vi "Batería electrónica (Main aplicación).vi"() -> ()   [LabVIEW 2015]
doc: "Este Vi contiene la máquina de estados necesaria para simular una batería electrónica, utilizando librerías DAQ y Arduino para recibir señales."
uses:
  <vilib>/DAQmx/read.llb/DAQmx Read (Analog DBL 1Chan 1Samp).vi
  <vilib>/DAQmx/create/channels.llb/DAQmx Create Channel (AI-Voltage-Basic).vi
  <vilib>/sound2/lvsound2.llb/Sound Output Write (DBL).vi
  <vilib>/DAQmx/miscellaneous.llb/DAQmx Fill In Error Info.vi
panel:
  in  "Stop Button":bool
  # "Batería Electrónica\nIICO UASLP"
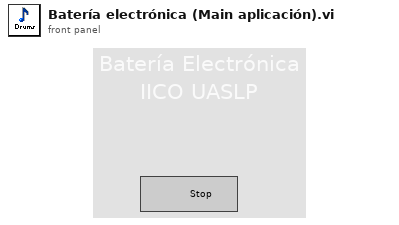
[diagram p1: front panel]
types:
  T1 = typedef "Control para máquina de estados.ctl" = enum16{"Bombo", "Medium Tom", "High Tom", "Hi-Hat ", "Tarola", "Tom de Piso", "Ride", "Crash"}
  T2 = typedef "Sound Output Task ID.ctl" = u32
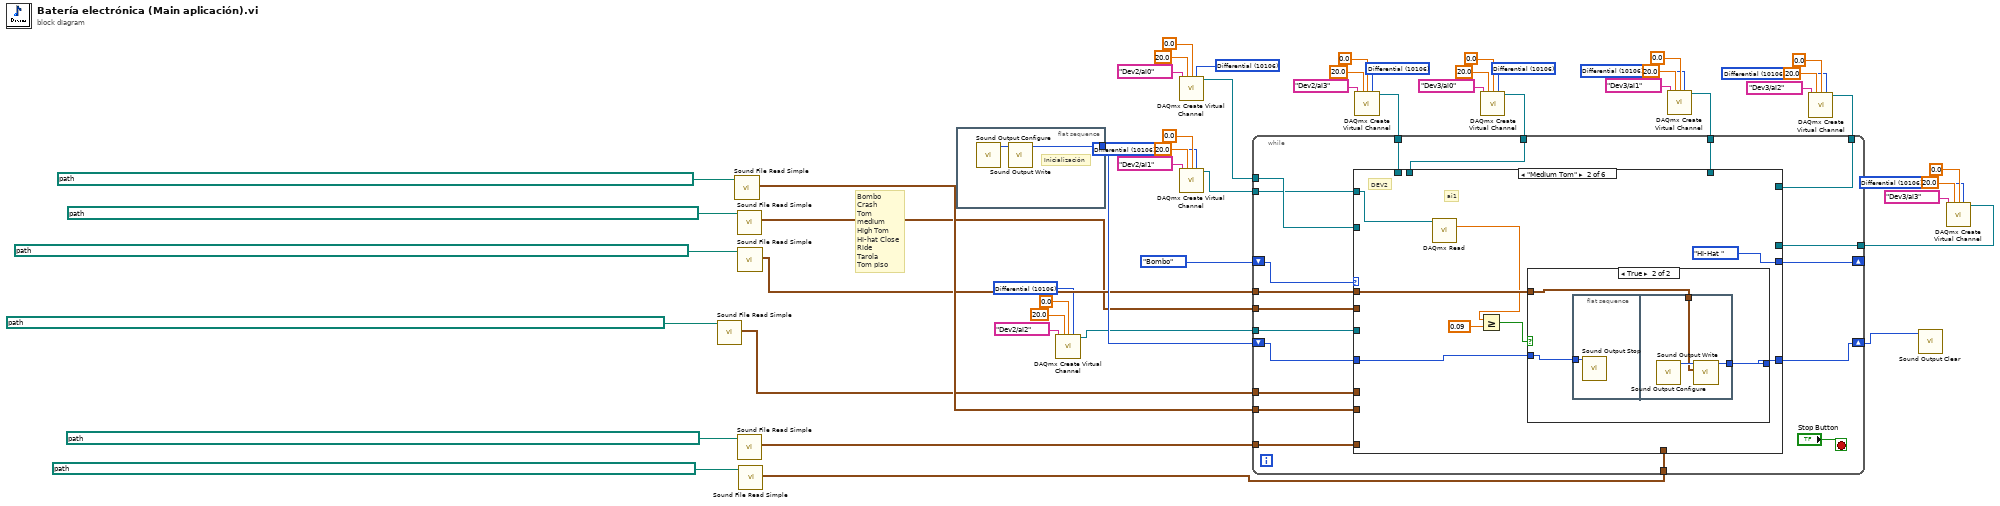
[diagram p0: block diagram]
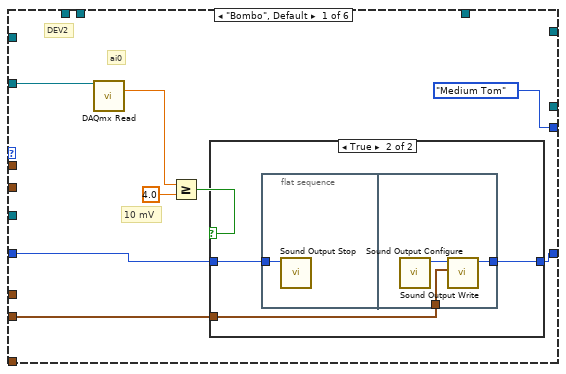
[diagram p2: hidden frame]
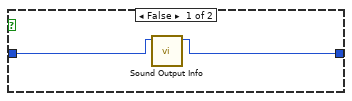
[diagram p3: hidden frame]
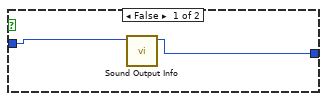
[diagram p4: hidden frame]
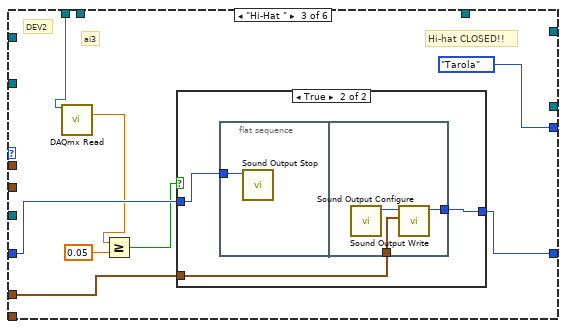
[diagram p5: hidden frame]
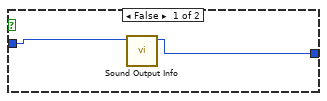
[diagram p6: hidden frame]
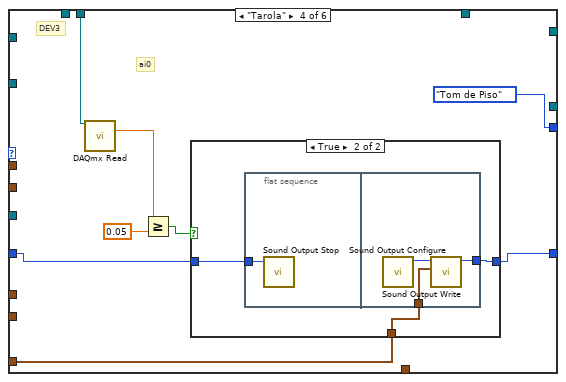
[diagram p7: hidden frame]
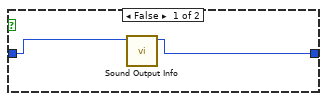
[diagram p8: hidden frame]
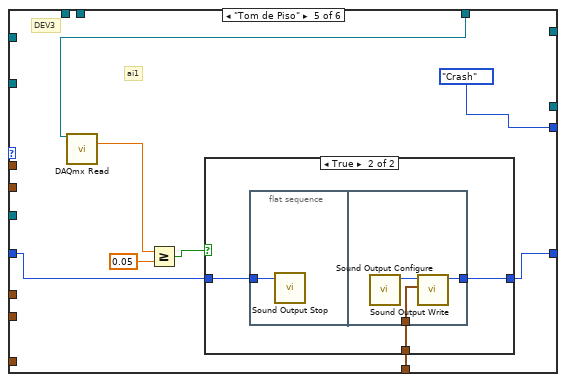
[diagram p9: hidden frame]
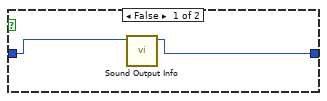
[diagram p10: hidden frame]
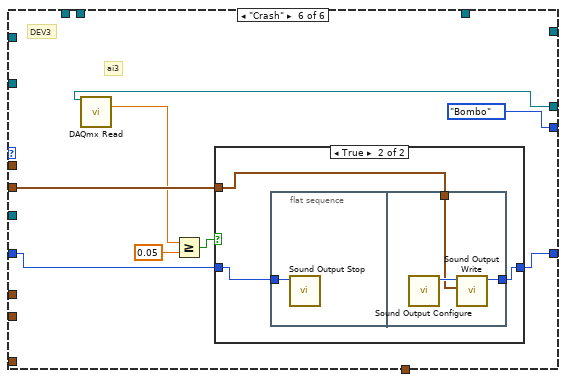
[diagram p11: hidden frame]
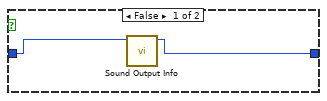
[diagram p12: hidden frame]
diagram:
  w2 = 10106 items=["Default"=-1, "RSE"=10083, "NRSE"=10078, "Differential"=10106, "Pseudodifferential"=12529] ("input terminal configuration")
  w6 = 10106 items=["Default"=-1, "RSE"=10083, "NRSE"=10078, "Differential"=10106, "Pseudodifferential"=12529] ("input terminal configuration")
  w8 = 10106 items=["Default"=-1, "RSE"=10083, "NRSE"=10078, "Differential"=10106, "Pseudodifferential"=12529] ("input terminal configuration")
  w13 = 10106 items=["Default"=-1, "RSE"=10083, "NRSE"=10078, "Differential"=10106, "Pseudodifferential"=12529] ("input terminal configuration")
  w18 = 10106 items=["Default"=-1, "RSE"=10083, "NRSE"=10078, "Differential"=10106, "Pseudodifferential"=12529] ("input terminal configuration")
  w22 = 10106 items=["Default"=-1, "RSE"=10083, "NRSE"=10078, "Differential"=10106, "Pseudodifferential"=12529] ("input terminal configuration")
  w23 = 10106 items=["Default"=-1, "RSE"=10083, "NRSE"=10078, "Differential"=10106, "Pseudodifferential"=12529] ("input terminal configuration")
  w24 = 10106 items=["Default"=-1, "RSE"=10083, "NRSE"=10078, "Differential"=10106, "Pseudodifferential"=12529] ("input terminal configuration")
  # "Bombo\nCrash\nTom medium\nHigh Tom\nHi-hat Close\nRide\nTarola\nTom piso"
  n1 = call <vilib>:"Sound File Read Simple.vi"("path"=path "C:/Users/user/Dropbox/INGENIERÍA FÍSICA/6to. Semestre/Laboratorio Ing Física 2 (Labview)/PROYECTO FINAL/Programa Final/seleccion final de samples/hi hat closed.wav") -> ("data"=w50:waveform(dbl)[])  [unwired: 7 in, 3 out]
  n2 = call <vilib>:"Sound File Read Simple.vi"("path"=path "C:/Users/user/Dropbox/INGENIERÍA FÍSICA/6to. Semestre/Laboratorio Ing Física 2 (Labview)/PROYECTO FINAL/Programa Final/seleccion final de samples/Bombo.wav") -> ("data"=w52:waveform(dbl)[])  [unwired: 7 in, 3 out]
  n3 = call <vilib>:"Sound File Read Simple.vi"("path"=path "C:/Users/user/Dropbox/INGENIERÍA FÍSICA/6to. Semestre/Laboratorio Ing Física 2 (Labview)/PROYECTO FINAL/Programa Final/seleccion final de samples/crash.wav") -> ("data"=w47:waveform(dbl)[])  [unwired: 7 in, 3 out]
  n4 = call <vilib>:"Sound File Read Simple.vi"("path"=path "C:/Users/user/Dropbox/INGENIERÍA FÍSICA/6to. Semestre/Laboratorio Ing Física 2 (Labview)/PROYECTO FINAL/Programa Final/seleccion final de samples/tarola.wav") -> ("data"=w49:waveform(dbl)[])  [unwired: 7 in, 3 out]
  n5 = call <vilib>:"Sound File Read Simple.vi"("path"=path "C:/Users/user/Dropbox/INGENIERÍA FÍSICA/6to. Semestre/Laboratorio Ing Física 2 (Labview)/PROYECTO FINAL/Programa Final/seleccion final de samples/tom medium final.wav") -> ("data"=w51:waveform(dbl)[])  [unwired: 7 in, 3 out]
  n6 = call <vilib>:"Sound File Read Simple.vi"("path"=path "C:/Users/user/Dropbox/INGENIERÍA FÍSICA/6to. Semestre/Laboratorio Ing Física 2 (Labview)/PROYECTO FINAL/Programa Final/seleccion final de samples/tom piso.wav") -> ("data"=w48:waveform(dbl)[])  [unwired: 7 in, 3 out]
  n7 = flat-sequence {
    tunnel: [w56] -> w54
    frame #0 {
      # "Inicialización"
      n8 = call <vilib>:"Sound Output Configure.vi"() -> ("task ID"=w57:T2)  [unwired: 10 in, 1 out]
      n9 = call-poly <vilib>:"Sound Output Write.vi"("task ID"=w57) -> ("task ID out"=w56:T2)  [unwired: 9 in, 1 out]
    }
  }
  n10 = call-poly <vilib>:"DAQmx Create Virtual Channel.vi"("maximum value"=20.0, "minimum value"=0.0, "input terminal configuration"=w6, "physical channels"=tag "Dev2/ai2") -> ("task out"=w29:refnum<k21>)  [unwired: 10 in, 1 out]
  n11 = call-poly <vilib>:"DAQmx Create Virtual Channel.vi"("maximum value"=20.0, "minimum value"=0.0, "input terminal configuration"=w23, "physical channels"=tag "Dev2/ai0") -> ("task out"=w39:refnum<k21>)  [unwired: 10 in, 1 out]
  n12 = call-poly <vilib>:"DAQmx Create Virtual Channel.vi"("maximum value"=20.0, "minimum value"=0.0, "input terminal configuration"=w22, "physical channels"=tag "Dev2/ai1") -> ("task out"=w33:refnum<k21>)  [unwired: 10 in, 1 out]
  n13 = call-poly <vilib>:"DAQmx Create Virtual Channel.vi"("maximum value"=20.0, "minimum value"=0.0, "input terminal configuration"=w24, "physical channels"=tag "Dev2/ai3") -> ("task out"=w25:refnum<k21>)  [unwired: 10 in, 1 out]
  n14 = call-poly <vilib>:"DAQmx Create Virtual Channel.vi"("maximum value"=20.0, "minimum value"=0.0, "input terminal configuration"=w18, "physical channels"=tag "Dev3/ai0") -> ("task out"=w17:refnum<k21>)  [unwired: 10 in, 1 out]
  n15 = call-poly <vilib>:"DAQmx Create Virtual Channel.vi"("maximum value"=20.0, "minimum value"=0.0, "input terminal configuration"=w13, "physical channels"=tag "Dev3/ai1") -> ("task out"=w12:refnum<k21>)  [unwired: 10 in, 1 out]
  n16 = call-poly <vilib>:"DAQmx Create Virtual Channel.vi"("maximum value"=20.0, "minimum value"=0.0, "input terminal configuration"=w8, "physical channels"=tag "Dev3/ai2") -> ("task out"=w7:refnum<k21>)  [unwired: 10 in, 1 out]
  n17 = call-poly <vilib>:"DAQmx Create Virtual Channel.vi"("maximum value"=20.0, "minimum value"=0.0, "input terminal configuration"=w2, "physical channels"=tag "Dev3/ai3") -> ("task out"=w1:refnum<k21>)  [unwired: 10 in, 1 out]
  n18 = while {
    shift-right: [w74] -> _
    shift-left: Control_para_máquina_de_estados."Bombo" -> [w75]
    shift-right: [w73] -> w53
    shift-left: w54 -> [w72]
    tunnel: w52 -> [w71]
    tunnel: w51 -> [w70]
    tunnel: w50 -> [w69]
    tunnel: w49 -> [w68]
    tunnel: w48 -> [w67]
    tunnel: w47 -> [w66]
    tunnel: w39 -> [w65]
    tunnel: w33 -> [w64]
    tunnel: w29 -> [w63]
    tunnel: w25 -> [w62]
    tunnel: w17 -> [w61]
    tunnel: w12 -> [w60]
    tunnel: w7 -> [w59]
    tunnel: w1 -> [w58]
    stop <- "Stop Button" stop-if-true
    n19 = case shown="\"Medium Tom\"" w75 {
      tunnel: [Control_para_máquina_de_estados."Medium Tom" Control_para_máquina_de_estados."Hi-Hat " Control_para_máquina_de_estados."Tarola" Control_para_máquina_de_estados."Tom de Piso" Control_para_máquina_de_estados."Crash" Control_para_máquina_de_estados."Bombo"] -> w74
      tunnel: [w83 w99 w114 w134 w150 w167] -> w73
      tunnel: w72 -> [w82 w100 w116 w133 w151 w168]
      tunnel: w71 -> [w81 _ _ _ _ _]
      tunnel: w70 -> [_ w98 _ _ _ _]
      tunnel: w69 -> [_ _ w113 _ _ _]
      tunnel: w68 -> [_ _ _ w132 _ _]
      tunnel: w67 -> [_ _ _ _ w149 _]
      tunnel: w66 -> [_ _ _ _ _ w166]
      tunnel: w65 -> [w78 _ _ _ _ _]
      tunnel: w64 -> [_ w94 _ _ _ _]
      tunnel: w63 -> [_ _ _ _ _ _]
      tunnel: w62 -> [_ _ w111 _ _ _]
      tunnel: w61 -> [_ _ _ w128 _ _]
      tunnel: w60 -> [_ _ _ _ w145 _]
      tunnel: w59 -> [_ _ _ _ _ _]
      tunnel: w58 -> [_ _ _ _ _ w163]
      frame "Bombo", Default {
        # "10 mV"
        # "DEV2"
        # "ai0"
        n20 = call-poly <vilib>:"DAQmx Read.vi"("task/channels in"=w78) -> ("data"=w77:dbl)  [unwired: 12 in, 2 out]
        n21 = Greater Or Equal?(x=w77, y=4.0) -> (x >= y?=w79:bool)
        n22 = case shown="True" w79 {
          tunnel: [w85 w89] -> w83
          tunnel: w82 -> [w86 w87]
          tunnel: w81 -> [_ w88]
          frame False {
            n23 = call <vilib>:"Sound Output Info.vi"("task ID"=w86) -> ("task ID out"=w85:T2)  [unwired: 7 in, 3 out]
          }
          frame True {
            n24 = flat-sequence {
              tunnel: w87 -> [w90]
              tunnel: [w92] -> w89
              tunnel: w88 -> [w91]
              frame #0 {
                n25 = call <vilib>:"Sound Output Stop.vi"("task ID"=w90) -> ()  [unwired: 9 in, 2 out]
              }
              frame #1 {
                n26 = call <vilib>:"Sound Output Configure.vi"() -> ("task ID"=w93:T2)  [unwired: 10 in, 1 out]
                n27 = call-poly <vilib>:"Sound Output Write.vi"("data"=w91, "task ID"=w93) -> ("task ID out"=w92:T2)  [unwired: 8 in, 1 out]
              }
            }
          }
        }
      }
      frame "Medium Tom" {
        # "DEV2"
        # "ai1"
        n28 = call-poly <vilib>:"DAQmx Read.vi"("task/channels in"=w94) -> ("data"=w95:dbl)  [unwired: 12 in, 2 out]
        n29 = Greater Or Equal?(x=w95, y=0.09) -> (x >= y?=w96:bool)
        n30 = case shown="True" w96 {
          tunnel: [w103 w106] -> w99
          tunnel: w100 -> [w102 w104]
          tunnel: w98 -> [_ w105]
          frame False {
            n31 = call <vilib>:"Sound Output Info.vi"("task ID"=w102) -> ("task ID out"=w103:T2)  [unwired: 7 in, 3 out]
          }
          frame True {
            n32 = flat-sequence {
              tunnel: w104 -> [w107]
              tunnel: [w109] -> w106
              tunnel: w105 -> [w108]
              frame #0 {
                n33 = call <vilib>:"Sound Output Stop.vi"("task ID"=w107) -> ()  [unwired: 9 in, 2 out]
              }
              frame #1 {
                n34 = call <vilib>:"Sound Output Configure.vi"() -> ("task ID"=w110:T2)  [unwired: 10 in, 1 out]
                n35 = call-poly <vilib>:"Sound Output Write.vi"("data"=w108, "task ID"=w110) -> ("task ID out"=w109:T2)  [unwired: 8 in, 1 out]
              }
            }
          }
        }
      }
      frame "Hi-Hat " {
        # "Hi-hat CLOSED!!"
        # "DEV2"
        # "ai3"
        n36 = call-poly <vilib>:"DAQmx Read.vi"("task/channels in"=w111) -> ("data"=w112:dbl)  [unwired: 12 in, 2 out]
        n37 = Greater Or Equal?(x=w112, y=0.05) -> (x >= y?=w115:bool)
        n38 = case shown="True" w115 {
          tunnel: [w120 w123] -> w114
          tunnel: w116 -> [w119 w121]
          tunnel: w113 -> [_ w122]
          frame False {
            n39 = call <vilib>:"Sound Output Info.vi"("task ID"=w119) -> ("task ID out"=w120:T2)  [unwired: 7 in, 3 out]
          }
          frame True {
            n40 = flat-sequence {
              tunnel: w121 -> [w124]
              tunnel: [w126] -> w123
              tunnel: w122 -> [w125]
              frame #0 {
                n41 = call <vilib>:"Sound Output Stop.vi"("task ID"=w124) -> ()  [unwired: 9 in, 2 out]
              }
              frame #1 {
                n42 = call <vilib>:"Sound Output Configure.vi"() -> ("task ID"=w127:T2)  [unwired: 10 in, 1 out]
                n43 = call-poly <vilib>:"Sound Output Write.vi"("data"=w125, "task ID"=w127) -> ("task ID out"=w126:T2)  [unwired: 8 in, 1 out]
              }
            }
          }
        }
      }
      frame "Tarola" {
        # "DEV3"
        # "ai0"
        n44 = call-poly <vilib>:"DAQmx Read.vi"("task/channels in"=w128) -> ("data"=w129:dbl)  [unwired: 12 in, 2 out]
        n45 = Greater Or Equal?(x=w129, y=0.05) -> (x >= y?=w130:bool)
        n46 = case shown="True" w130 {
          tunnel: [w137 w140] -> w134
          tunnel: w133 -> [w136 w138]
          tunnel: w132 -> [_ w139]
          frame False {
            n47 = call <vilib>:"Sound Output Info.vi"("task ID"=w136) -> ("task ID out"=w137:T2)  [unwired: 7 in, 3 out]
          }
          frame True {
            n48 = flat-sequence {
              tunnel: w138 -> [w141]
              tunnel: [w143] -> w140
              tunnel: w139 -> [w142]
              frame #0 {
                n49 = call <vilib>:"Sound Output Stop.vi"("task ID"=w141) -> ()  [unwired: 9 in, 2 out]
              }
              frame #1 {
                n50 = call <vilib>:"Sound Output Configure.vi"() -> ("task ID"=w144:T2)  [unwired: 10 in, 1 out]
                n51 = call-poly <vilib>:"Sound Output Write.vi"("data"=w142, "task ID"=w144) -> ("task ID out"=w143:T2)  [unwired: 8 in, 1 out]
              }
            }
          }
        }
      }
      frame "Tom de Piso" {
        # "DEV3"
        # "ai1"
        n52 = call-poly <vilib>:"DAQmx Read.vi"("task/channels in"=w145) -> ("data"=w146:dbl)  [unwired: 12 in, 2 out]
        n53 = Greater Or Equal?(x=w146, y=0.05) -> (x >= y?=w147:bool)
        n54 = case shown="True" w147 {
          tunnel: [w154 w157] -> w150
          tunnel: w151 -> [w153 w155]
          tunnel: w149 -> [_ w156]
          frame False {
            n55 = call <vilib>:"Sound Output Info.vi"("task ID"=w153) -> ("task ID out"=w154:T2)  [unwired: 7 in, 3 out]
          }
          frame True {
            n56 = flat-sequence {
              tunnel: w155 -> [w158]
              tunnel: [w160] -> w157
              tunnel: w156 -> [w159]
              frame #0 {
                n57 = call <vilib>:"Sound Output Stop.vi"("task ID"=w158) -> ()  [unwired: 9 in, 2 out]
              }
              frame #1 {
                n58 = call <vilib>:"Sound Output Configure.vi"() -> ("task ID"=w161:T2)  [unwired: 10 in, 1 out]
                n59 = call-poly <vilib>:"Sound Output Write.vi"("data"=w159, "task ID"=w161) -> ("task ID out"=w160:T2)  [unwired: 8 in, 1 out]
              }
            }
          }
        }
      }
      frame "Crash" {
        # "ai3"
        # "DEV3"
        n60 = call-poly <vilib>:"DAQmx Read.vi"("task/channels in"=w163) -> ("data"=w162:dbl)  [unwired: 12 in, 2 out]
        n61 = Greater Or Equal?(x=w162, y=0.05) -> (x >= y?=w164:bool)
        n62 = case shown="True" w164 {
          tunnel: [w171 w174] -> w167
          tunnel: w168 -> [w170 w172]
          tunnel: w166 -> [_ w173]
          frame False {
            n63 = call <vilib>:"Sound Output Info.vi"("task ID"=w170) -> ("task ID out"=w171:T2)  [unwired: 7 in, 3 out]
          }
          frame True {
            n64 = flat-sequence {
              tunnel: w172 -> [w175]
              tunnel: [w177] -> w174
              tunnel: w173 -> [w176]
              frame #0 {
                n65 = call <vilib>:"Sound Output Stop.vi"("task ID"=w175) -> ()  [unwired: 9 in, 2 out]
              }
              frame #1 {
                n66 = call <vilib>:"Sound Output Configure.vi"() -> ("task ID"=w178:T2)  [unwired: 10 in, 1 out]
                n67 = call-poly <vilib>:"Sound Output Write.vi"("data"=w176, "task ID"=w178) -> ("task ID out"=w177:T2)  [unwired: 8 in, 1 out]
              }
            }
          }
        }
      }
    }
  }
  n68 = call <vilib>:"Sound Output Clear.vi"("task ID"=w53) -> ()  [unwired: 10 in, 1 out]
